vi "Read Filter_Wheel.lvclass.vi"(8 "error in (no error)":errorcluster, 11 "SPARC4_GEI in":refnum<class "SPARC4_GEI.lvclass">) -> (0 "error out":errorcluster, 2 "Filter_Wheel.lvclass":refnum<class "Filter_Wheel.lvclass">, 3 "SPARC4_GEI out":refnum<class "SPARC4_GEI.lvclass">)   [LabVIEW 2018, in "SPARC4_GEI.lvclass"]
uses:
  SPARC4_GEI.lvclass
  Filter_Wheel/Filter_Wheel.lvclass
  SPARC4_GEI.lvclass/SPARC4_GEI.ctl
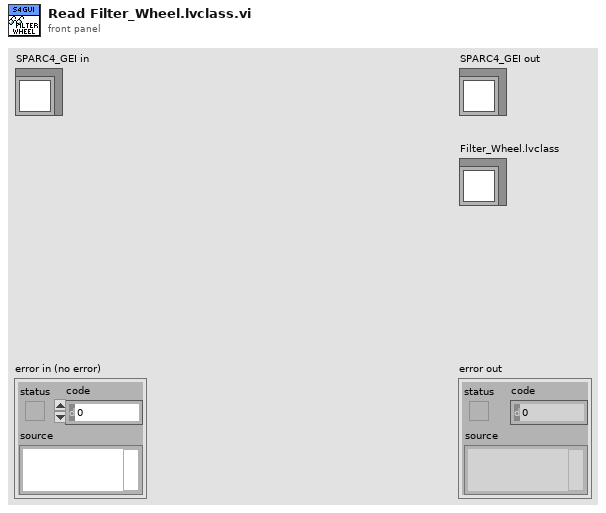
[diagram p1: front panel]
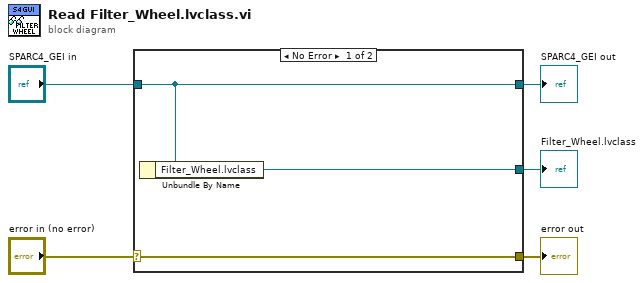
[diagram p0: block diagram]
diagram:
  n1 = case shown="No Error" "error in (no error)" {
    selector: "error in (no error)" -> [w8 w9]
    tunnel: [w8 w9] -> w4
    tunnel: [w7 w10] -> w2
    tunnel: "SPARC4_GEI in" -> [w7 w10]
    tunnel: [w6 _] -> w1
    frame No Error {
      n2 = Unbundle By Name(w7) -> ("Filter_Wheel.lvclass"=w6:refnum<class "Filter_Wheel.lvclass">)
    }
    frame Error {
    }
  }
  "error out" <- w4
  "SPARC4_GEI out" <- w2
  "Filter_Wheel.lvclass" <- w1
